vi "ArduinoToLabVIEW- Prediction.vi"(11 "reference":refnum<visa-resource-name>) -> (0 "SD":dbl, 3 "VISA resource name out":refnum<visa-resource-name>)   [LabVIEW 2021]
panel:
  out "before substring":string
  out "concatenated string":string
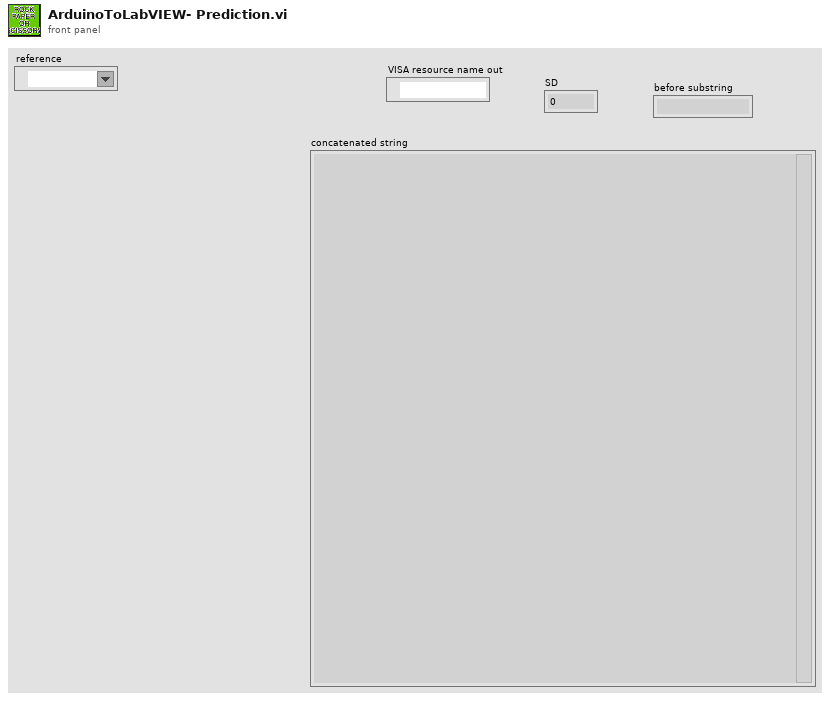
[diagram p1: front panel]
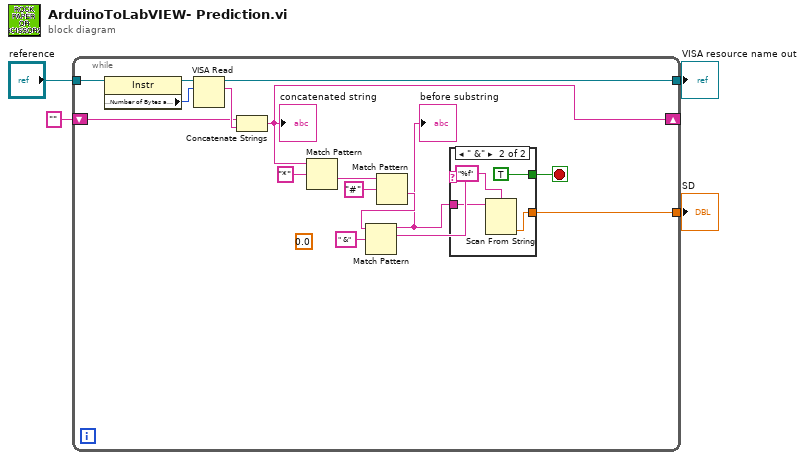
[diagram p0: block diagram]
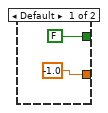
[diagram p2: hidden frame]
diagram:
  n1 = while {
    tunnel: "reference" -> [w14]
    shift-right: [w11] -> _
    shift-left: "" -> [w13]
    tunnel: [w10] -> w3
    tunnel: [w12] -> w2
    stop <- w9 stop-if-true
    (unwired) 0.0
    n2 = property class="Instr"(reference=w14) -> (reference out=w15:refnum<visa-resource-name>, "Serial Settings:Number of Bytes at Serial Port"=w16:u32)  [unwired: 1 in, 1 out]
    n3 = VISA Read(VISA resource name=w15, byte count=w16) -> (VISA resource name out=w12:refnum<visa-resource-name>, read buffer=w17:string)  [unwired: 1 in, 2 out]
    n4 = Concatenate Strings(w13, w17) -> (w11:string)
    "concatenated string" <- w11
    n5 = Match Pattern(string=w11, regular expression="*") -> (after substring=w20:string)  [unwired: 1 in, 3 out]
    n6 = Match Pattern(string=w20, regular expression="#") -> (after substring=w8:string)  [unwired: 1 in, 3 out]
    n7 = Match Pattern(string=w8, regular expression=" &") -> (before substring=w5:string, match substring=w6:string)  [unwired: 1 in, 2 out]
    "before substring" <- w5
    n8 = case shown="\" &\"" w6 {
      tunnel: [-1.0 w23] -> w10
      tunnel: [FALSE TRUE] -> w9
      tunnel: w5 -> [_ w24]
      frame Default {
      }
      frame " &" {
        n9 = Scan From String(format string="%f", input string=w24) -> (output 1=w23:dbl)  [unwired: 3 in, 3 out]
      }
    }
  }
  "SD" <- w3
  "VISA resource name out" <- w2
